vi "3d Test2.vi"() -> ()   [LabVIEW 2017]
uses:
  <vilib>/picture/3D Picture Control/Object/Create Object (name).vi
  <vilib>/picture/3D Picture Control/Object/Create Object (drawable).vi
  <vilib>/picture/3D Picture Control/Object/Add Object (reference).vi
  <vilib>/picture/3D Picture Control/NI_3D Picture Control.lvlib
panel:
  out "3D Picture":refnum<vi>(3d-picture)
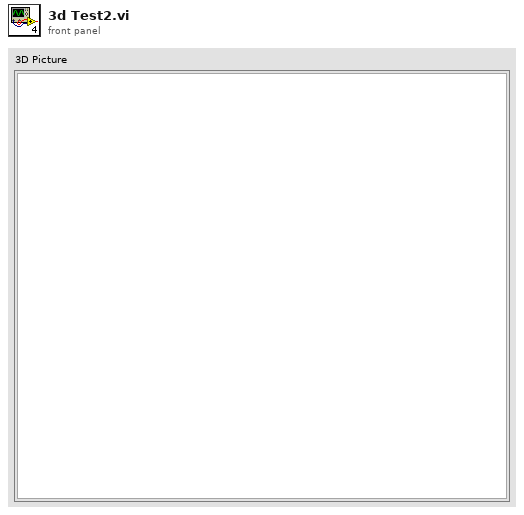
[diagram p1: front panel]
types:
  T1 = cluster{"Red":sgl, "Green":sgl, "Blue":sgl, "Alpha":sgl}
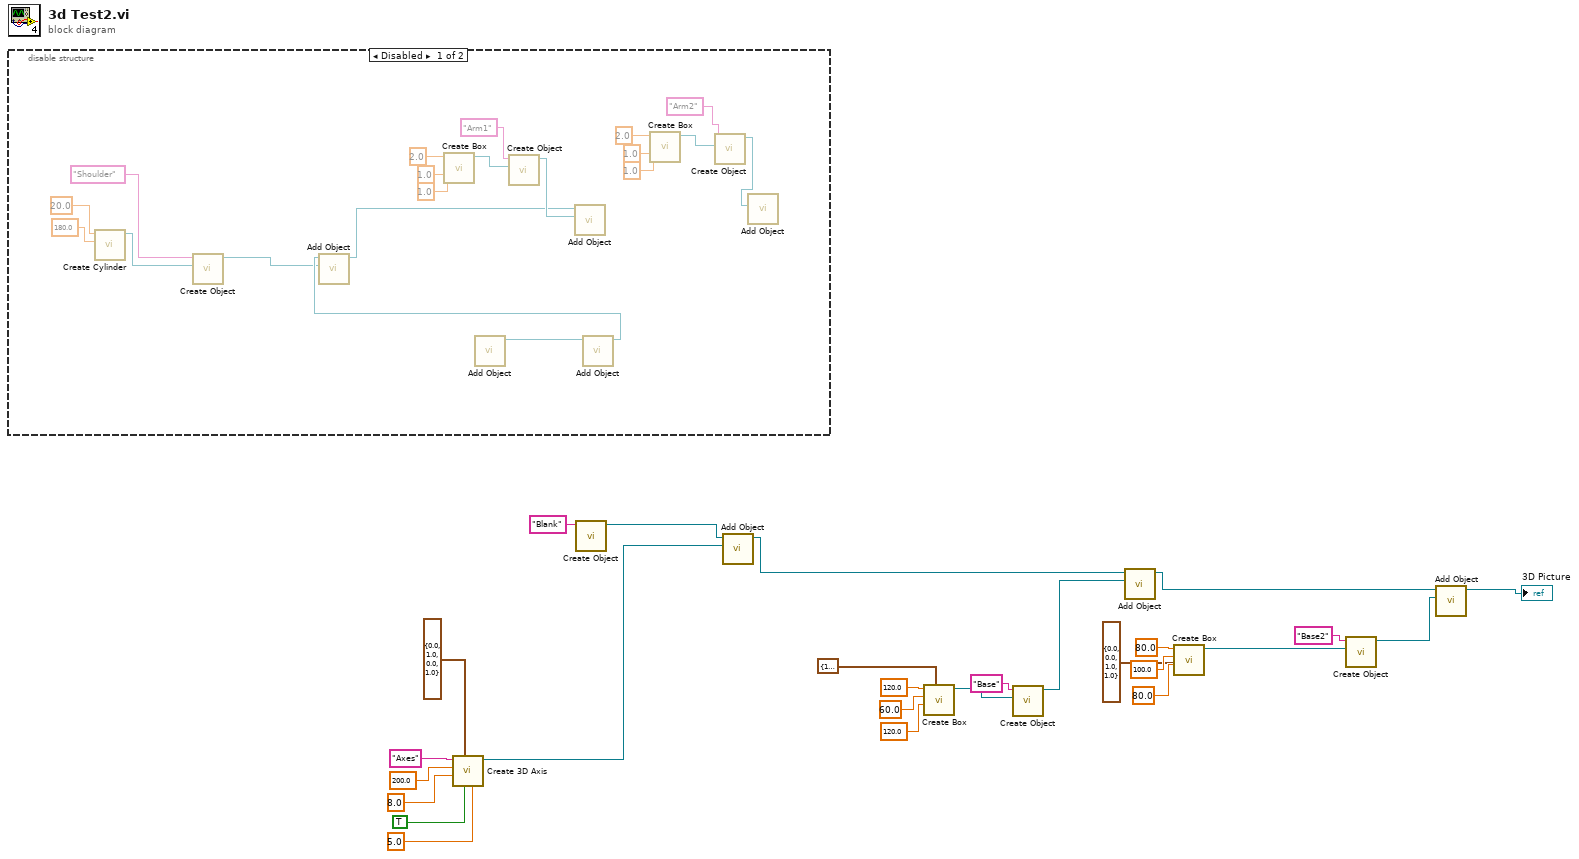
[diagram p0: block diagram]
diagram:
  n1 = disable-structure shown="Disabled" {
    frame Disabled {
      n2 = call <vilib>:"Create Cylinder.vi"("Radius"=sgl 180.0 ("Length Y"), "Height"=sgl 20.0 ("Length X")) -> ("New Cylinder Refnum"=w42:refnum<vi>)  [unwired: 8 in, 1 out]
      n3 = call-poly <vilib>:"Create Object.vi"("Geometry"=w42, "Name"="Shoulder") -> ("Scene:New Object"=w37:refnum<vi>)  [unwired: 8 in, 1 out]
      n4 = call <vilib>:"Create Box.vi"("Length Z"=sgl 1.0, "Length Y"=sgl 1.0, "Length X"=sgl 2.0) -> ("New Box Refnum"=w44:refnum<vi>)  [unwired: 7 in, 1 out]
      n5 = call-poly <vilib>:"Add Object.vi"() -> ("Scene Object Out"=w39:refnum<vi>)  [unwired: 9 in, 2 out]
      n6 = call-poly <vilib>:"Create Object.vi"("Geometry"=w44, "Name"="Arm1") -> ("Scene:New Object"=w28:refnum<vi>)  [unwired: 8 in, 1 out]
      n7 = call-poly <vilib>:"Add Object.vi"("Scene Object In"=w39) -> ("Scene Object Out"=w38:refnum<vi>)  [unwired: 8 in, 2 out]
      n8 = call-poly <vilib>:"Add Object.vi"("New Object In"=w37, "Scene Object In"=w38) -> ("Scene Object Out"=w27:refnum<vi>)  [unwired: 7 in, 2 out]
      n9 = call-poly <vilib>:"Add Object.vi"("New Object In"=w28, "Scene Object In"=w27) -> ()  [unwired: 7 in, 3 out]
      n10 = call <vilib>:"Create Box.vi"("Length Z"=sgl 1.0, "Length Y"=sgl 1.0, "Length X"=sgl 2.0) -> ("New Box Refnum"=w32:refnum<vi>)  [unwired: 7 in, 1 out]
      n11 = call-poly <vilib>:"Create Object.vi"("Geometry"=w32, "Name"="Arm2") -> ("Scene:New Object"=w29:refnum<vi>)  [unwired: 8 in, 1 out]
      n12 = call-poly <vilib>:"Add Object.vi"("New Object In"=w29) -> ()  [unwired: 8 in, 3 out]
    }
    frame Enabled {
    }
  }
  n13 = call <vilib>:"Create 3D Axis.vi"("Character Size"=sgl 5.0, "Axis label?"=TRUE, "Color"=T1 {"Red"=0.0, "Green"=1.0, "Blue"=0.0, "Alpha"=1.0}, "Radius"=sgl 8.0, "Length"=sgl 200.0, "Name"="Axes") -> ("New Object Refnum"=w2:refnum<vi>)  [unwired: 4 in, 1 out]
  n14 = call-poly <vilib>:"Create Object.vi"("Name"="Blank") -> ("Scene:New Object"=w9:refnum<vi>)  [unwired: 9 in, 1 out]
  n15 = call-poly <vilib>:"Add Object.vi"("New Object In"=w2, "Scene Object In"=w9) -> ("Scene Object Out"=w1:refnum<vi>)  [unwired: 7 in, 2 out]
  n16 = call <vilib>:"Create Box.vi"("Color"=T1 {"Red"=1.0, "Green"=0.0, "Blue"=1.0, "Alpha"=1.0}, "Length Z"=sgl 120.0, "Length Y"=sgl 60.0, "Length X"=sgl 120.0) -> ("New Box Refnum"=w23:refnum<vi>)  [unwired: 6 in, 1 out]
  n17 = call-poly <vilib>:"Create Object.vi"("Geometry"=w23, "Name"="Base") -> ("Scene:New Object"=w19:refnum<vi>)  [unwired: 8 in, 1 out]
  n18 = call-poly <vilib>:"Add Object.vi"("New Object In"=w19, "Scene Object In"=w1) -> ("Scene Object Out"=w12:refnum<vi>)  [unwired: 7 in, 2 out]
  n19 = call <vilib>:"Create Box.vi"("Color"=T1 {"Red"=0.0, "Green"=0.0, "Blue"=1.0, "Alpha"=1.0}, "Length Z"=sgl 80.0, "Length Y"=sgl 100.0, "Length X"=sgl 80.0) -> ("New Box Refnum"=w17:refnum<vi>)  [unwired: 6 in, 1 out]
  n20 = call-poly <vilib>:"Create Object.vi"("Geometry"=w17, "Name"="Base2") -> ("Scene:New Object"=w11:refnum<vi>)  [unwired: 8 in, 1 out]
  n21 = call-poly <vilib>:"Add Object.vi"("New Object In"=w11, "Scene Object In"=w12) -> ("Scene Object Out"=→"3D Picture":refnum<vi>)  [unwired: 7 in, 2 out]
